vi "Inset Direction.vi"(8 "error in (no error)":errorcluster, 10 "Keyboard":T1, 11 "Board_Game in":refnum<class "Board_Game.lvclass">) -> (0 "error out":errorcluster, 3 "Board_Game out":refnum<class "Board_Game.lvclass">)   [LabVIEW 2021, in "Board_Game.lvclass"]
uses:
  Board_Game.lvclass
  Direction.ctl
  Board_Game.lvclass/Board_Game.ctl
  SnakeGame/Snake.lvclass
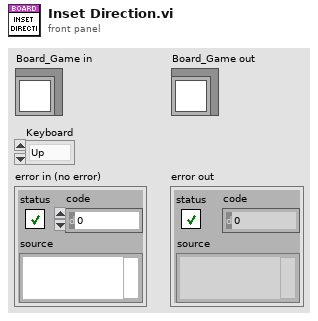
[diagram p1: front panel]
types:
  T1 = typedef "Direction.ctl" = enum16{"Up", "Down", "Left", "Right"}
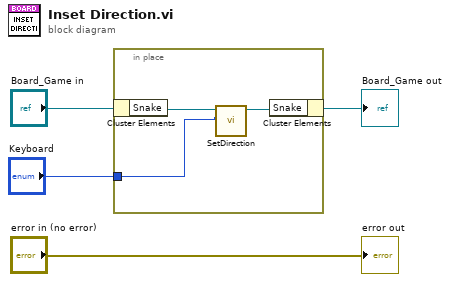
[diagram p0: block diagram]
diagram:
  n1 = in-place {
    in-place-border: "Keyboard" -> [w6]
    n2 = in-place-cluster #1("Board_Game in") -> ("Snake"=w7:refnum<class "Snake.lvclass">)
    n3 = call-dynamic "SetDirection.vi"("Direction"=w6, "Snake in"=w7) -> ("Snake out"=w5:refnum<class "Snake.lvclass">)  [unwired: 8 in, 1 out]
    n4 = in-place-cluster #1("Snake"=w5) -> (→"Board_Game out":refnum<class "Board_Game.lvclass">)
  }
  "error out" <- "error in (no error)"
